vi "MinerConnectServer.vi"(0 "HostIP":string="149.91.88.18", 1 "远程端口或服务名称":u16=6004) -> (3 "connection ID out":refnum<k5>, 4 "版本号":string="2.4", 5 "Good":bool, 6 "错误输出 2":errorcluster caption="错误输出")   [LabVIEW 2014]
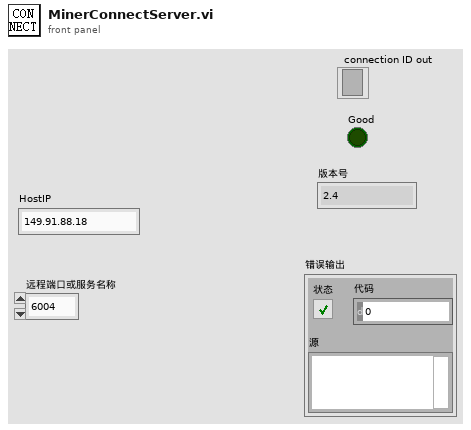
[diagram p1: front panel]
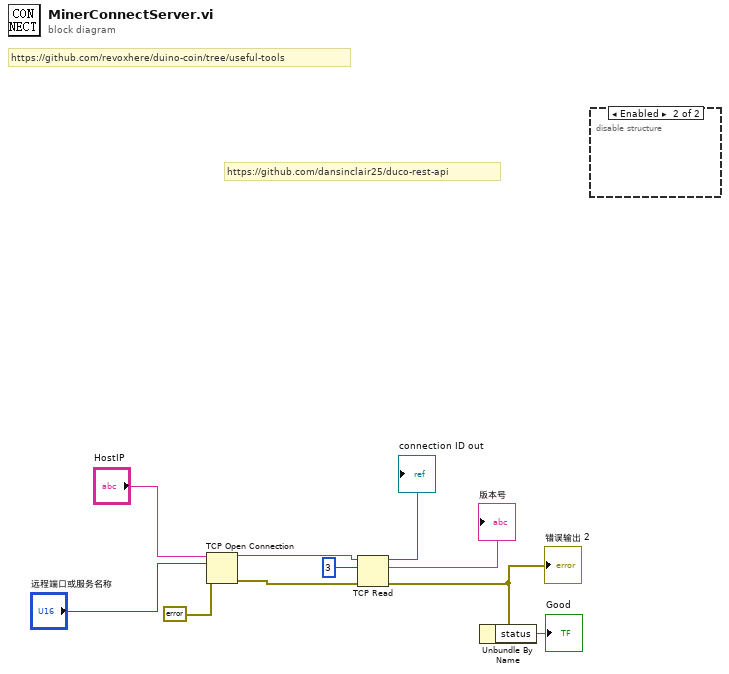
[diagram p0: block diagram]
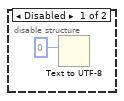
[diagram p2: hidden frame]
diagram:
  # "https://github.com/dansinclair25/duco-rest-api"
  # "https://github.com/revoxhere/duino-coin/tree/useful-tools"
  n1 = TCP Open Connection(address="HostIP", remote port or service name="远程端口或服务名称", error in (no error)=errorcluster {"status"=FALSE, "code"=0, "source"=""} ("错误输入（无错误）")) -> (connection ID=w10:refnum<k5>, error out=w9:errorcluster)  [unwired: 2 in]
  n2 = TCP Read(connection ID=w10, bytes to read=3 ("读取的字节"), error in (no error)=w9) -> (connection ID out=→"connection ID out":refnum<k5>, data out=→"版本号":string, error out=w3:errorcluster)  [unwired: 2 in]
  "错误输出 2" <- w3
  n3 = Unbundle By Name(w3) -> ("status"=→"Good":bool)
  n4 = disable-structure shown="Enabled" {
    frame Disabled {
      n5 = Text to UTF-8(10:0 ("编码（系统默认=-1）")) -> ()  [unwired: 2 in, 2 out]
    }
    frame Enabled {
    }
  }
